vi "New Instance.vi"(8 "error in":errorcluster) -> (0 "error out":errorcluster, 3 "GLue out":refnum<class "class.GLue.lvclass">)   [LabVIEW 2014, in "GLue.lvlib"]
doc: "Creates a new instance of GLue which can be wired to other GLue API functions.\n\n<B>Parameter(s) </B>\n-----------------\n\n- <B>error in:</B> Describes error conditions that occur before this node runs. This input provides standard error in functionality. \n\n- <B>GLue out:</B> Newly created GLue instance.\n\n- <B>error out:</B> Contains error information. This output provides standard error out functionality."
uses:
  GLue.lvlib
  Private/Class/class.GLue.lvclass
panel:
  # "Input"
  # "Output"
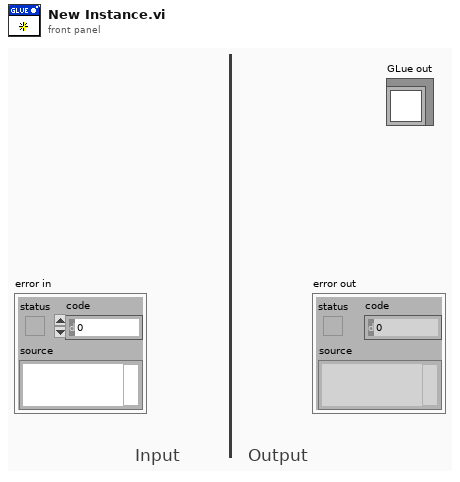
[diagram p1: front panel]
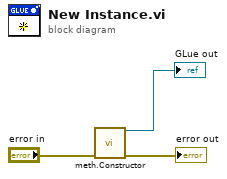
[diagram p0: block diagram]
diagram:
  n1 = call "meth.Constructor.vi"("error in"="error in") -> ("GLue out"=→"GLue out":refnum<class "class.GLue.lvclass">, "error out"=→"error out":errorcluster)  [unwired: 13 in]
